vi "Release.vi"(8 "error in (no error)":errorcluster, 11 "MessageQ in":refnum<class "MessageQ.lvclass">) -> (0 "error out":errorcluster)   [LabVIEW 2020, in "Volatus.lvlib" / "MessageQ.lvclass"]
uses:
  MessageQ.lvclass
  MessageQ.lvclass/MessageQ.ctl
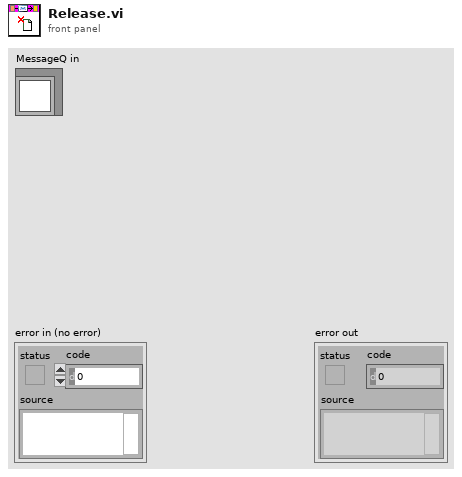
[diagram p1: front panel]
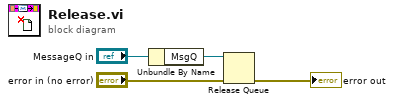
[diagram p0: block diagram]
diagram:
  n1 = Unbundle By Name("MessageQ in") -> ("MsgQ"=w3:refnum<queue>)
  n2 = Release Queue(queue=w3, error in (no error)="error in (no error)") -> (error out=→"error out":errorcluster)  [unwired: 1 in, 2 out]
